vi "Using VRML with File.vi"() -> ()   [LabVIEW 2023]
doc: "Demonstrates how to load a model from a .wrl file into a 3D Picture with the Load VRML File VI."
uses:
  <vilib>/picture/3D Picture Control/NI_3D Picture Control.lvlib
panel:
  in  "Apply Changes":bool
  in  "Stop":bool
  in  "VRML String":string="#VRML V2.0 utf8\n#Stealth Bomber\n\n#body 1\nDEF body1\nTransform { \n   scale .8, 1, .5\n   translation 0,1,0\n   children [\n     Shape {\n      appearance Appearance {\n         material Material {\n        diffuseColor .7 .7 .7}      }\n      geometry Cone {\n           height 1\n           bottomRadius .5} \n       } ] } # end geometry-children-transform\n\n#body 2\nDEF body2\nTransform { \n   scale .8, 1, .5\n   translation 0,-.85,0\n   rotation 1,0,0,3.14\n   children [\n     Shape {\n      appearance Appearance {\n         material Material {\n        diffuseColor .7 .7 .7} \n       }\n      geometry Cone {\n           height 2.7\n           bottomRadius .5} \n       }  ] }\n\nDEF wing1\nTransform {\n  scale 4.6, 1.1, .05\n  children [\n    Shape {\n      appearance Appearance {\n        material Material {\n          diffuseColor .7 .7 .7 }   }\n      geometry Cone {\n        height 2.5\n        bottomRadius .5 }\n    }  ]  }\n\nDEF wingtip1\nTransform {\n  translation 1.95,-1.5,0\n  rotation 0,0,1,.69\n  children [\n    Shape {\n      appearance Appearance {\n        material Material {\n          diffuseColor .7 .7 .7\n        } \n      }\n      geometry Box {\n        size .7 1 .01    } \n    }  ]  }\n\nDEF wingtip2\nTransform {\n  translation -1.95,-1.5,0\n  rotation 0,0,1,-.69\n  children [\n    Shape {\n      appearance Appearance {\n        material Material {\n          diffuseColor .7 .7 .7 }  }\n      geometry Box {\n        size .7 1 .01 } \n     } ] }\n\nDEF wingtip3\nTransform {\n  translation -.9,-1.2,0\n  rotation 0,0,1,.9\n  children [\n    Shape {\n      appearance Appearance {\n        material Material {\n          diffuseColor .7 .7 .7 }  }\n      geometry Box {\n        size .8 1.5 .01 }\n    }  ] }\n\nDEF wingtip4\nTransform {\n  translation .9,-1.2,0\n  rotation 0,0,1,-.9\n  children [\n    Shape {\n      appearance Appearance {\n        material Material {\n          diffuseColor .7 .7 .7 }  }\n      geometry Box {\n        size .8 1.5 .01 }\n    }  ] }\n\nDEF cockpit\nTransform{\n  translation 0, .65, .1\n  scale 1.2, 3, 1\n  children [\n    Shape {\n      appearance Appearance {\n        material Material {\n          diffuseColor .5 .5 1 } } \n      geometry Sphere {\n        radius .16  } \n    } ] } "
  out "3D Picture":refnum<vi>(3d-picture)
  # "Overview: Demonstrates how to load a model from a temporary .wrl file into a 3D Picture with the Load VRML File VI.\nRequirements: LabVIEW Full Development System\nInstructions:\n1. Run the VI. The model contained in the VRML String below will be displayed in the 3D Picture.\n2. Modify the VRML String and click Apply Changes. If you specified valid VRML, the new image will be displayed. If you specified invalid VRML, the VI will generate an error.\n3. Click Stop to stop the VI."
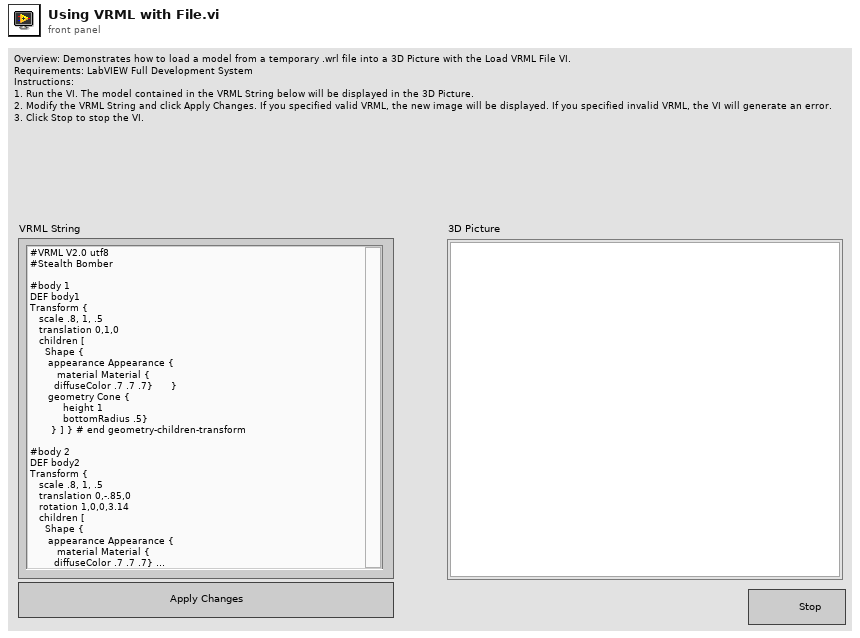
[diagram p1: front panel]
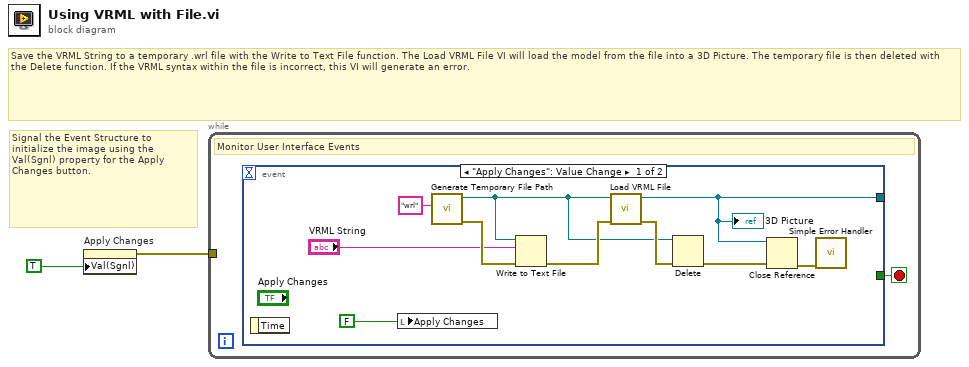
[diagram p0: block diagram]
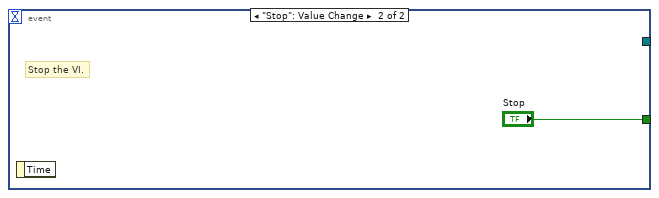
[diagram p2: hidden frame]
diagram:
  # "Signal the Event Structure to initialize the image using the Val(Sgnl) property for the Apply Changes button."
  # "Save the VRML String to a temporary .wrl file with the Write to Text File function. The Load VRML File VI will load the model from the file into a 3D Picture. The temporary file is then deleted with the Delete function. If the VRML syntax within the file is incorrect, this VI will generate an error."
  n1 = property on="Apply Changes" class="Bool (strict)"("Val(Sgnl)"=TRUE ("Value (Signaling)")) -> (error out=w2:errorcluster)  [unwired: 2 in, 1 out]
  n2 = while {
    tunnel: w2 -> [_]
    stop <- w3 stop-if-true
    # "Monitor User Interface Events"
    n3 = event shown="[0] \"Apply Changes\": Value Change" {
      selector: _ -> [_ _]
      dyn-events: _ -> [_ _]
      timeout: _ -> [_ _]
      tunnel: [w5 _] -> _
      tunnel: [_ "Stop"] -> w3
      event "Apply Changes": Value Change {
        n4 = event-data() -> ()  [unwired: 1 in, 1 out]
        n5 = local write "Apply Changes"(FALSE ("Apply Changes")) -> ()
        n6 = call <vilib>:"Generate Temporary File Path.vi"("Temporary File Extension (tmp)"="wrl") -> ("error out"=w11:errorcluster, "Unique Temporary File Path"=w9:path)  [unwired: 9 in]
        n7 = Write to Text File(file (use dialog)=w9, text="VRML String", error in=w11) -> (error out=w10:errorcluster)  [unwired: 1 in, 2 out]
        n8 = call <vilib>:"Load VRML File.vi"("error in"=w10, "Path"=w9) -> ("error out"=w13:errorcluster, "Scene:Read Scene File"=w5:refnum<vi>)  [unwired: 8 in]
        "3D Picture" <- w5
        n9 = Delete(path (use dialog)=w9, error in=w13) -> (error out=w6:errorcluster)  [unwired: 3 in, 2 out]
        n10 = Close Reference(reference=w5, error in (no error)=w6) -> (error out=w4:errorcluster)
        n11 = call <vilib>:"Simple Error Handler.vi"("error in (no error)"=w4) -> ()  [unwired: 4 in, 5 out]
      }
      event "Stop": Value Change {
        # "Stop the VI."
        n12 = event-data() -> ()  [unwired: 1 in, 1 out]
      }
    }
  }
